vi "Agilent34401AMeasure.vi"(8 "error in (no error)":errorcluster) -> (0 "error out":errorcluster, 3 "Measurement":dbl)   [LabVIEW 2014]
uses:
  FGV.ctl
  <instrlib>/Agilent 34401/Public/Data/Read (Single Point).vi
  <instrlib>/Agilent 34401/Agilent 34401.lvlib
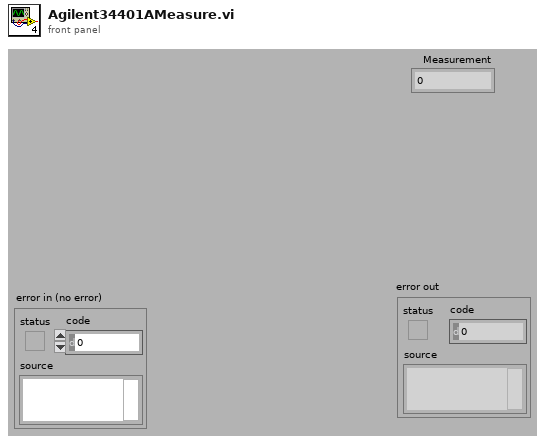
[diagram p1: front panel]
types:
  T1 = typedef "FGV.ctl" = enum16{"Write", "Read", "Init"}
  T2 = typedef "Agilent34401AData.ctl" = cluster{"Adress":refnum<visa-resource-name>}
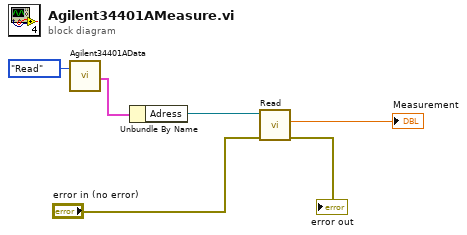
[diagram p0: block diagram]
diagram:
  n1 = call "Agilent34401AData.vi"("Enum"=FGV."Read") -> ("Cluster 2"=w5:T2)  [unwired: 17 in, 1 out]
  n2 = Unbundle By Name(w5) -> ("Adress"=w2:refnum<visa-resource-name>)
  n3 = call-poly <instrlib>:"Read.vi"("error in (no error)"="error in (no error)", "VISA resource name"=w2) -> ("error out"=→"error out":errorcluster, "Measurement"=→"Measurement":dbl)  [unwired: 7 in, 1 out]
